vi "Problem 13 - Large sum.vi"() -> ()   [LabVIEW 2021, in "Project Euler.lvlib"]
uses:
  Project Euler.lvlib
  Utilities/Named Timers/Named Timers.lvlib
panel:
  in  "no. of elements to generate":i32=100
  in  "element":string="123456789\n"
  out "Test input":string
  out "Answer: first ten digits of sum":string
  out "first column (last iteration)":string
  out "first column (last iteration)":i32
  out "sum: number of digits":i32
  out "sum":string
  out "no. of digits per number":i32
  out "no. of numbers":i32
  out "2D array\nEach row is a number (50 columns)\nEach cell is a digit of a number":string[][](array[string])
  out "no. of numbers":i32
  out "100 x 50 digit numbers (one element for each number)":string[](array[string])
  in  "100 x 50-digit numbers":string="37107287533902102798797998220837590246510135740250\n46376937677490009712648124896970078050417018260538\n74324986199524741059474233309513058123726617309629\n91942213363574161572522430563301811072406154908250\n23067588207539346171171980310421047513778063246676\n89261670696623633820136378418383684178734361726757\n28112879812849979408065481931592621691275889832738\n44274228917432520321923589422876796487670272189318\n47451445736001306439091167216856844588711603153276\n70386486105843025439939619828917593665686757934951\n62176457141856560629502157223196586755079324193331\n649063524627419049291014324458138226633..."
  out "Total execution time (ms)":u32
  # "Development\nControls or indicators that are useful for development or testing, but which are not outputs of the VI."
  # "Input\nInputs to the VI"
  # "Output\nOutputs of the VI"
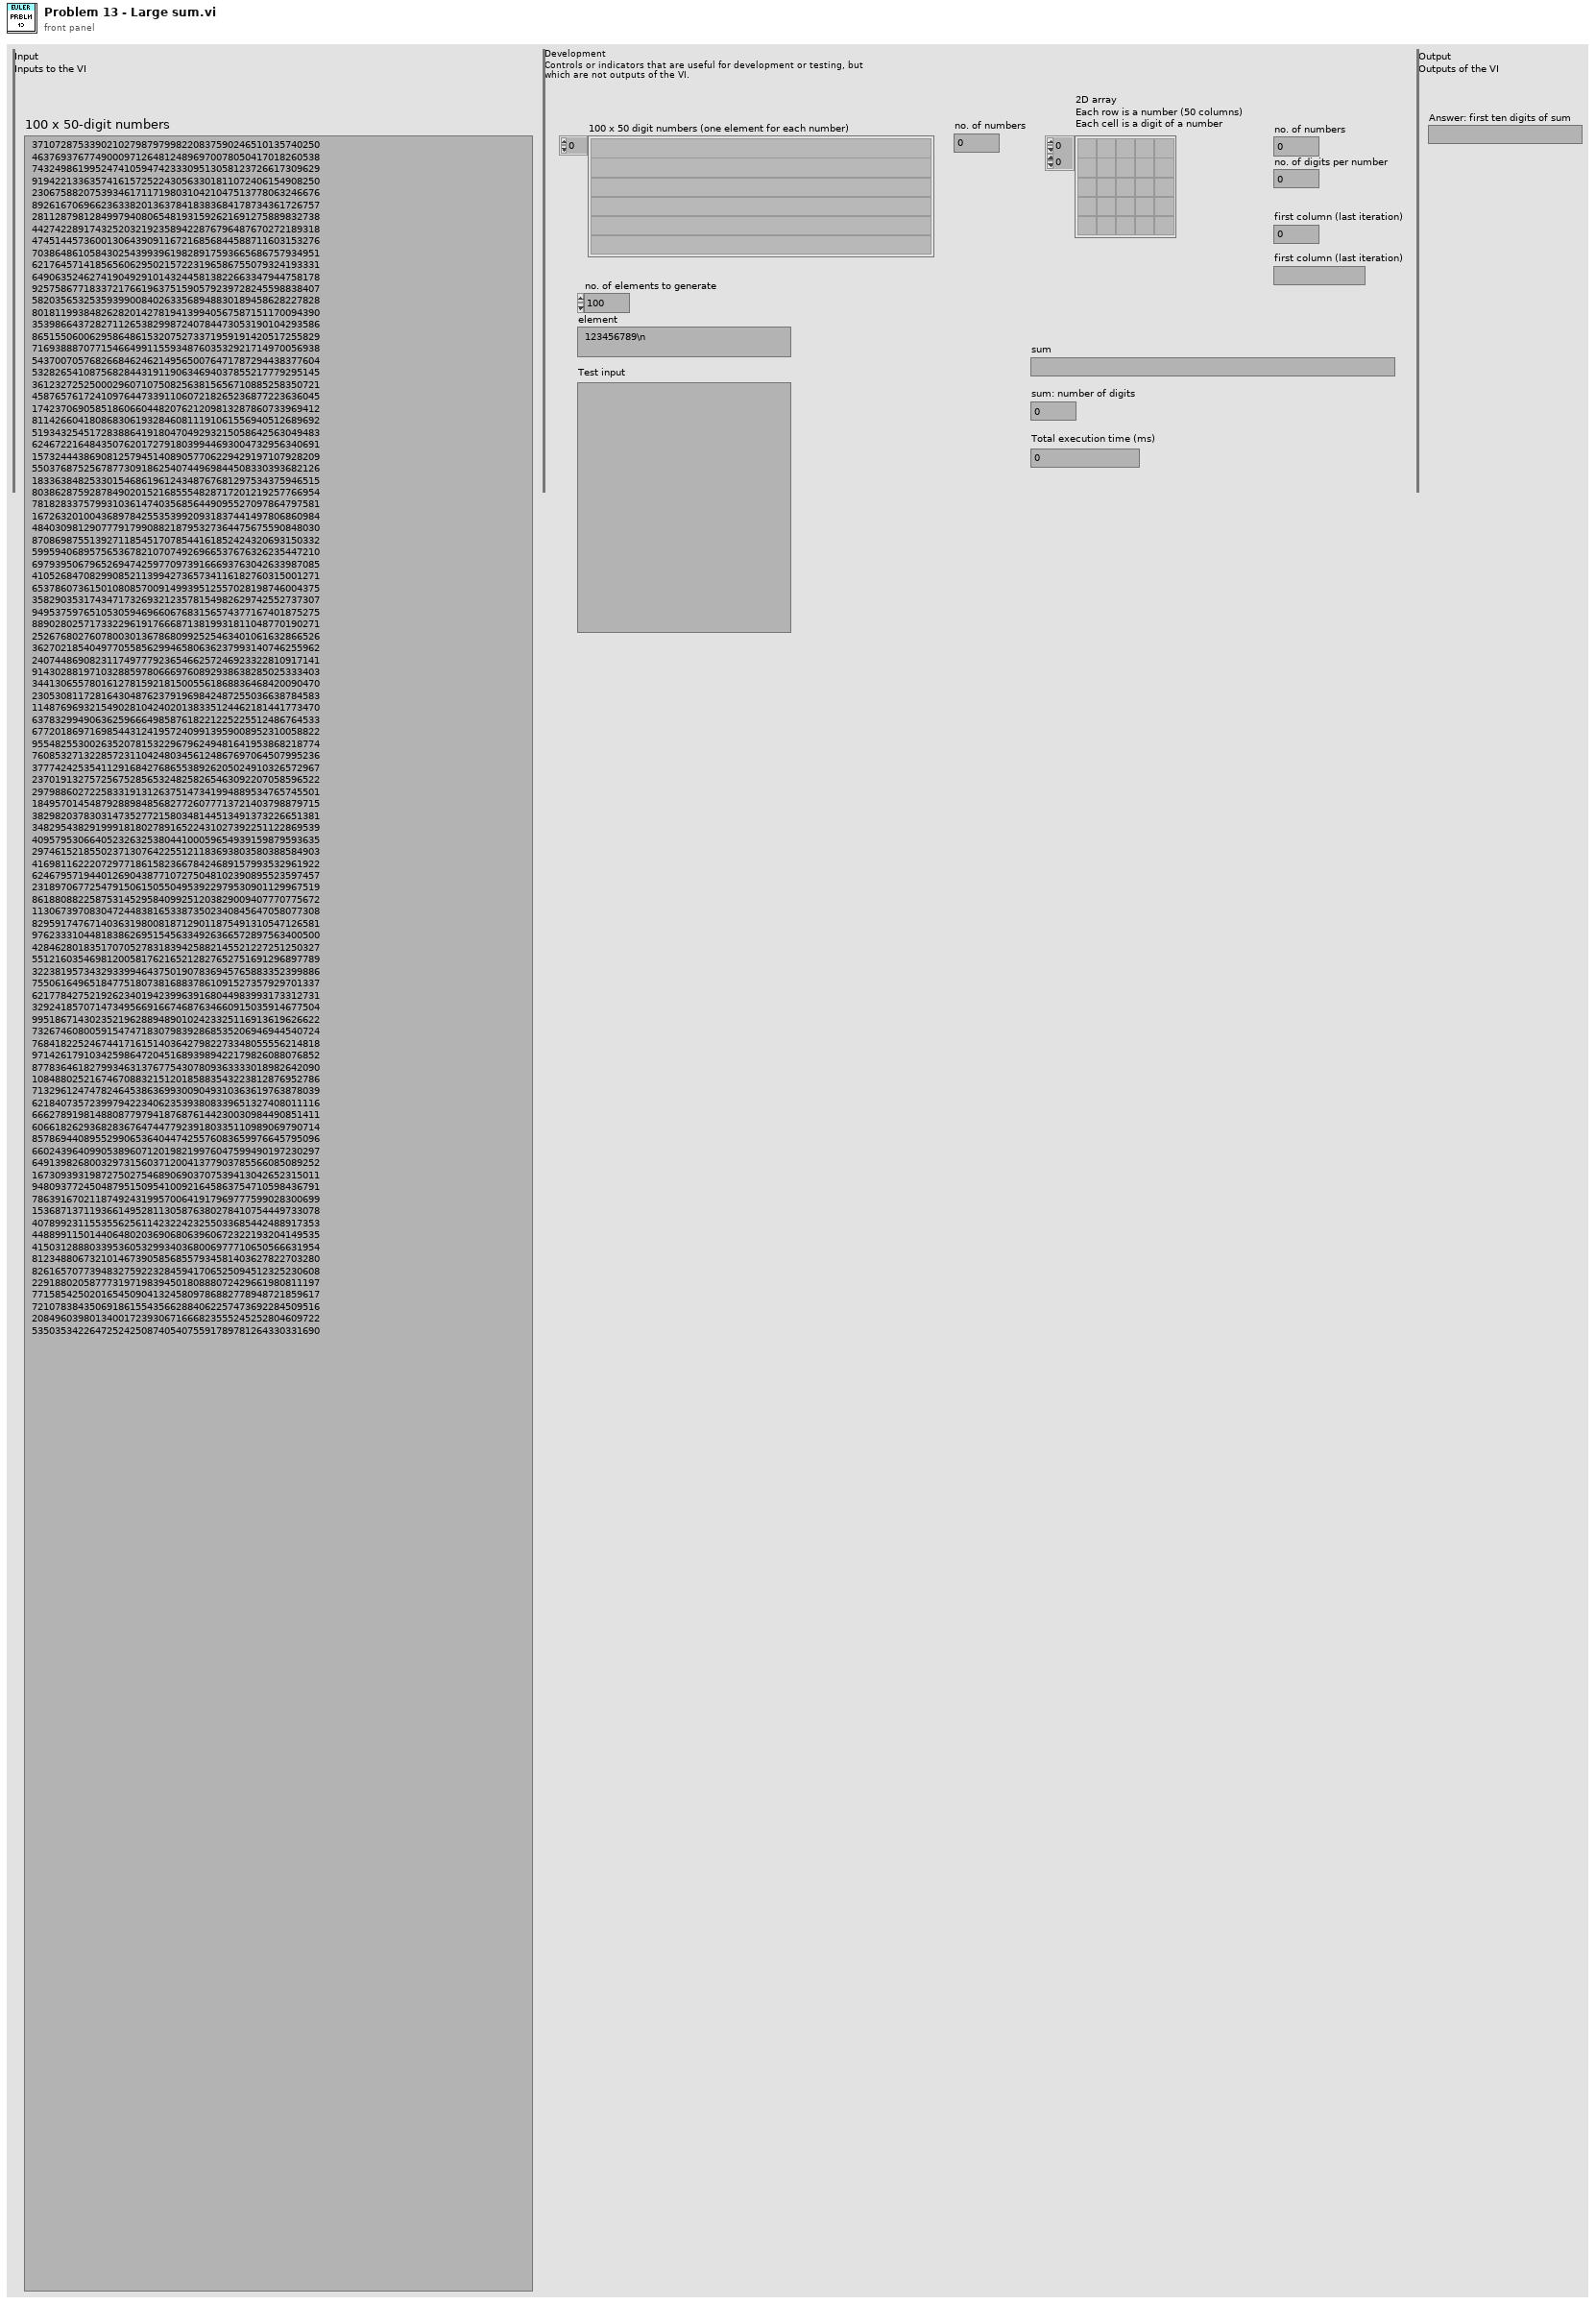
[diagram p1: front panel]
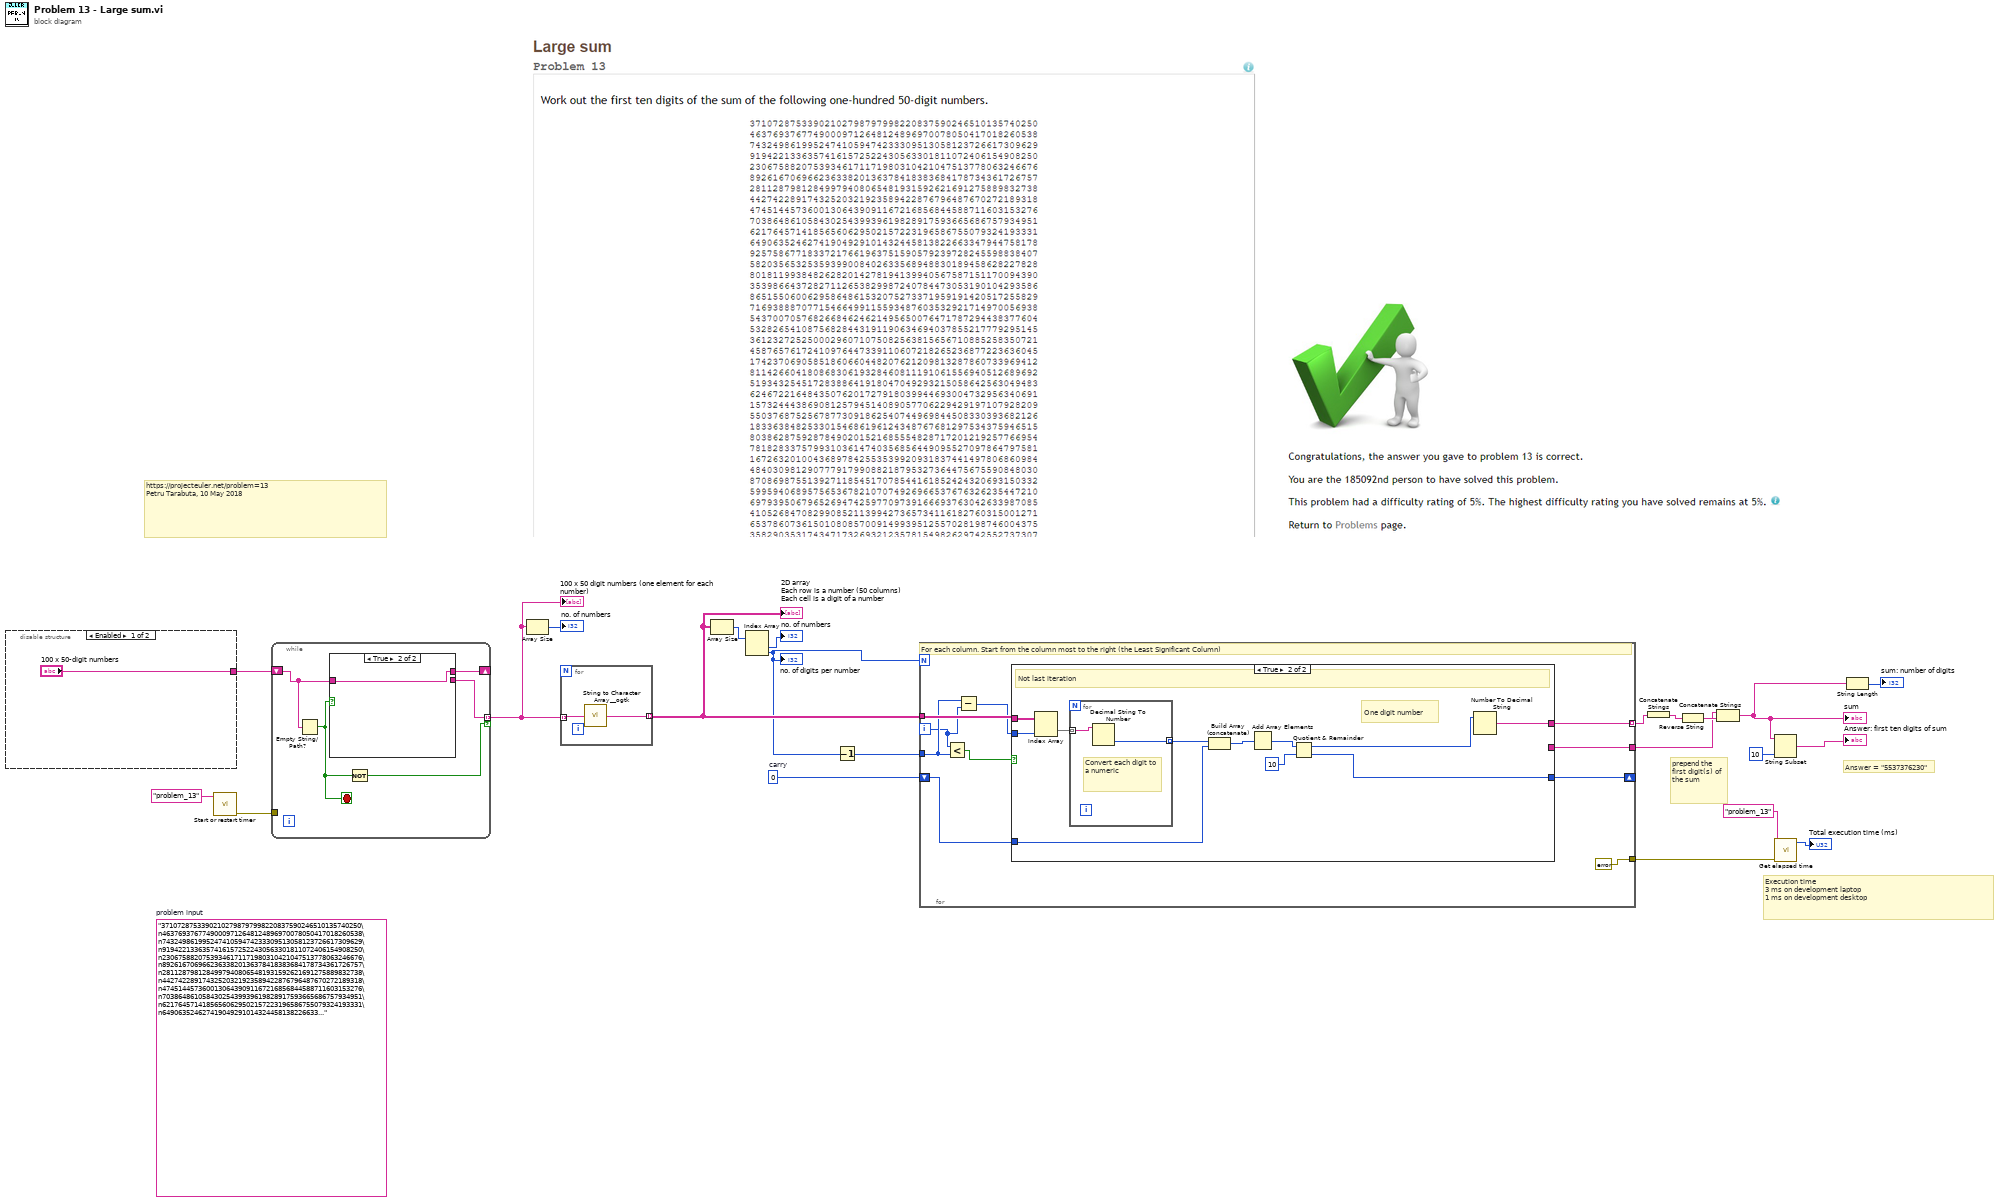
[diagram p0: block diagram]
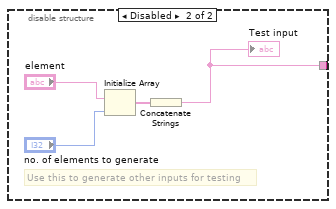
[diagram p2: hidden frame]
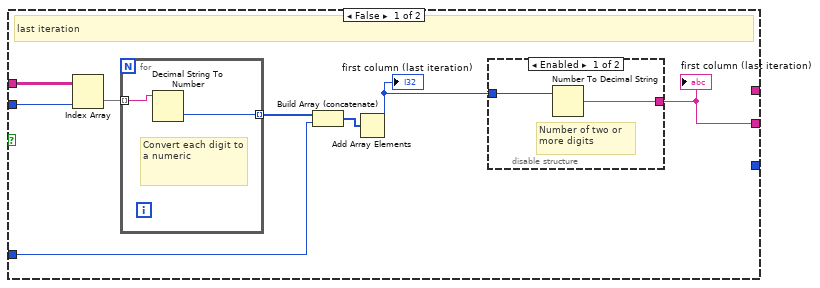
[diagram p3: hidden frame]
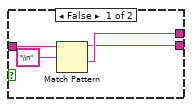
[diagram p5: hidden frame]
diagram:
  (unwired) "37107287533902102798797998220837590246510135740250\n46376937677490009712648124896970078050417018260538\n74324986199524741059474233309513058123726617309629\n91942213363574161572522430563301811072406154908250\n23067588207539346171171980310421047513778063246676\n89261670696623633820136378418383684178734361726757\n28112879812849979408065481931592621691275889832738\n44274228917432520321923589422876796487670272189318\n47451445736001306439091167216856844588711603153276\n70386486105843025439939619828917593665686757934951\n62176457141856560629502157223196586755079324193331\n649063524627419049291014324458138226633..."  # problem input
  w14 = 0  # carry
  # "Answer = \"5537376230\""
  # "prepend the first digit(s) of the sum"
  # "Execution time\n3 ms on development laptop\n1 ms on development desktop"
  # "https://projecteuler.net/problem=13\nPetru Tarabuta, 10 May 2018"
  n1 = disable-structure shown="Enabled" {
    disable-tunnel: ["100 x 50-digit numbers" w24] -> w20
    frame Enabled {
    }
    frame Disabled {
      # "Use this to generate other inputs for testing"
      n2 = Initialize Array("element", "no. of elements to generate") -> (w27:string[])
      n3 = Concatenate Strings(w27) -> (w24:string)
      "Test input" <- w24
    }
  }
  n4 = call "Start or restart timer.vi"("Timer name"="problem_13") -> ("error out"=w2:errorcluster)  [unwired: 10 in]
  n5 = while {
    shift-right: [w32] -> _
    shift-left: w20 -> [w31]
    tunnel: [w28] -> w18 mode=indexing if=w30
    tunnel: w2 -> [_]
    stop <- w29 stop-if-true
    n6 = Empty String/Path?(string/path=w31) -> (empty?=w29:bool)
    n7 = case shown="True" w29 {
      tunnel: [w35 w37] -> w32
      tunnel: w31 -> [w34 w37]
      tunnel: [w33 _] -> w28
      frame False {
        n8 = Match Pattern(string=w34, regular expression="\\n") -> (before substring=w33:string, after substring=w35:string)  [unwired: 1 in, 2 out]
      }
      frame True {
      }
    }
    n9 = Not(x=w29) -> (.not. x?=w30:bool)
  }
  "100 x 50 digit numbers (one element for each number)" <- w18
  n10 = Array Size(array=w18) -> (size(s)=→"no. of numbers":i32)
  n11 = for {
    tunnel: w18 -> [w39] mode=indexing
    tunnel: [w38] -> w15 mode=indexing
    n12 = call <userlib>:"String to Character Array__ogtk.vi"("Input String"=w39) -> ("Character Array"=w38:string[])
  }
  "2D array\nEach row is a number (50 columns)\nEach cell is a digit of a number" <- w15
  n13 = Array Size(array=w15) -> (size(s)=w17:i32[])
  n14 = Index Array(array=w17) -> (element #1=→"no. of numbers":i32, element #2=w10:i32)  [unwired: 2 in]
  "no. of digits per number" <- w10
  n15 = Decrement(x=w10) -> (x-1=w8:i32)
  n16 = for {
    N: w10 -> [_]
    tunnel: w15 -> [w49]
    shift-right: [w48] -> _
    shift-left: w14 -> [w47]
    tunnel: [w46] -> w13 mode=indexing
    tunnel: w8 -> [w42]
    tunnel: [w44] -> w7
    tunnel: [errorcluster {"status"=FALSE, "code"=0, "source"=""} ("error constant")] -> w1
    i -> [w41]
    # "For each column. Start from the column most to the right (the Least Significant Column)"
    n17 = Less?(x=w41, y=w42) -> (x < y?=w45:bool)
    n18 = Subtract(x=w42, y=w41) -> (x-y=w40:i32)
    n19 = case shown="True" w45 {
      tunnel: w49 -> [w55 w72]
      tunnel: [_ w68] -> w48
      tunnel: w47 -> [w52 w66]
      tunnel: [_ w64] -> w46
      tunnel: w40 -> [w54 w63]
      tunnel: [w50 _] -> w44
      frame False {
        # "last iteration"
        n20 = Index Array(array=w55, index (col)=w54) -> (element=w56:string[])  [unwired: 1 in]
        n21 = for {
          tunnel: w56 -> [w61] mode=indexing
          tunnel: [w60] -> w57 mode=indexing
          # "Convert each digit to a numeric"
          n22 = Decimal String To Number(string=w61) -> (number=w60:i32)  [unwired: 2 in, 1 out]
        }
        n23 = Build Array (concatenate)(w57, w52) -> (w53:i32[])
        n24 = Add Array Elements(numeric array=w53) -> (sum=w51:i32)
        "first column (last iteration)" <- w51
        n25 = disable-structure shown="Enabled" {
          disable-tunnel: [w59 _] -> w50
          disable-tunnel: w51 -> [w58 _]
          frame Enabled {
            # "Number of two or more digits"
            n26 = Number To Decimal String(number=w58) -> (decimal integer string=w59:string)  [unwired: 1 in]
          }
          frame Disabled {
          }
        }
        "first column (last iteration)" <- w50
      }
      frame True {
        # "One digit number"
        # "Not last iteration"
        n27 = Index Array(array=w72, index (col)=w63) -> (element=w62:string[])  [unwired: 1 in]
        n28 = for {
          tunnel: w62 -> [w74] mode=indexing
          tunnel: [w73] -> w71 mode=indexing
          # "Convert each digit to a numeric"
          n29 = Decimal String To Number(string=w74) -> (number=w73:i32)  [unwired: 2 in, 1 out]
        }
        n30 = Build Array (concatenate)(w71, w66) -> (w67:i32[])
        n31 = Add Array Elements(numeric array=w67) -> (sum=w70:i32)
        n32 = Quotient & Remainder(x=w70, y=10) -> (x-y*floor(x/y)=w65:i32, floor(x/y)=w68:i32)
        n33 = Number To Decimal String(number=w65) -> (decimal integer string=w64:string)  [unwired: 1 in]
      }
    }
  }
  n34 = Concatenate Strings(w13) -> (w12:string)
  n35 = Reverse String(1:w12) -> (0:w9:string)
  n36 = Concatenate Strings(w7, w9) -> (w6:string)
  "sum" <- w6
  n37 = String Subset(string=w6, length (rest)=10 ("length (rest)")) -> (substring=→"Answer: first ten digits of sum":string)  [unwired: 1 in]
  n38 = call "Get elapsed time.vi"("error in (no error)"=w1, "Timer name"="problem_13") -> ("Elapsed time (ms)"=→"Total execution time (ms)":u32)  [unwired: 6 in, 3 out]
  n39 = String Length(string=w6) -> (length=→"sum: number of digits":i32)
